vi "dayode.vi"() -> ()   [LabVIEW 2020]
uses:
  <vilib>/Analysis/baseanly.llb/Mean (DBL).vi
  <vilib>/Analysis/NI_AALBase.lvlib
panel:
  out "x-y":dbl
  out "led 2":bool
  in  "stop":bool
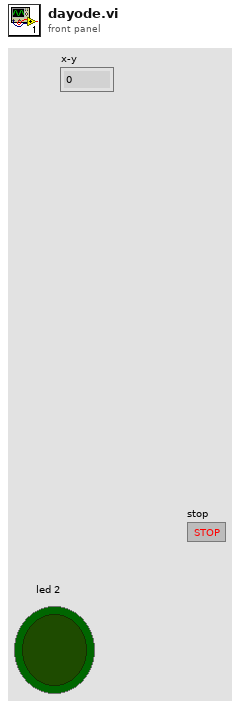
[diagram p1: front panel]
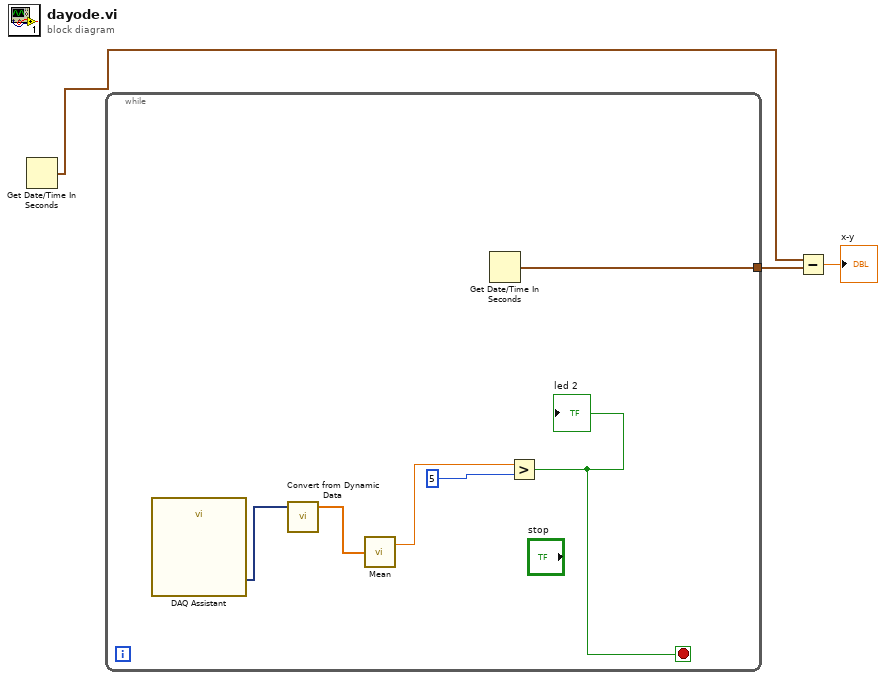
[diagram p0: block diagram]
diagram:
  n1 = Get Date/Time In Seconds() -> (seconds since 1Jan1904=w3:timestamp)
  n2 = while {
    tunnel: [w4] -> w2
    stop <- w5 stop-if-true
    n3 = call "DAQ Assistant"() -> ("data"=w8:dynamicdata)  [unwired: 17 in, 2 out]
    n4 = call "Convert from Dynamic Data"("Dynamic Data Type"=w8) -> ("Array"=w7:dbl[])  [unwired: 3 in]
    n5 = call-poly <vilib>:"Mean.vi"("X"=w7) -> ("mean"=w6:dbl)  [unwired: 1 out]
    n6 = Get Date/Time In Seconds() -> (seconds since 1Jan1904=w4:timestamp)
    n7 = Greater?(x=w6, y=5) -> (0:w5:bool)
    "led 2" <- w5
  }
  n8 = Subtract(x=w3, y=w2) -> (x-y=→"x-y":dbl)
